vi "Create.vi"(8 "error in (no error)":errorcluster) -> (0 "error out":errorcluster, 3 "String Argument Matching Comparator":refnum<class "Matching String Input Comparator.lvclass">)   [LabVIEW 2020, in "Matching String Input Comparator.lvclass"]
uses:
  Matching String Input Comparator.lvclass
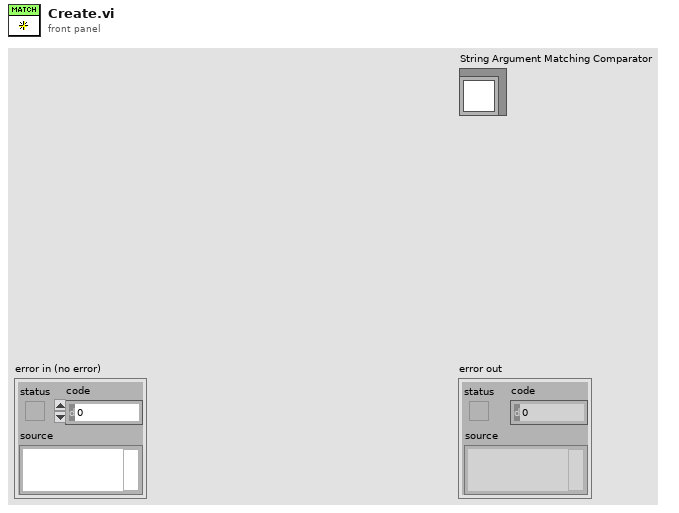
[diagram p1: front panel]
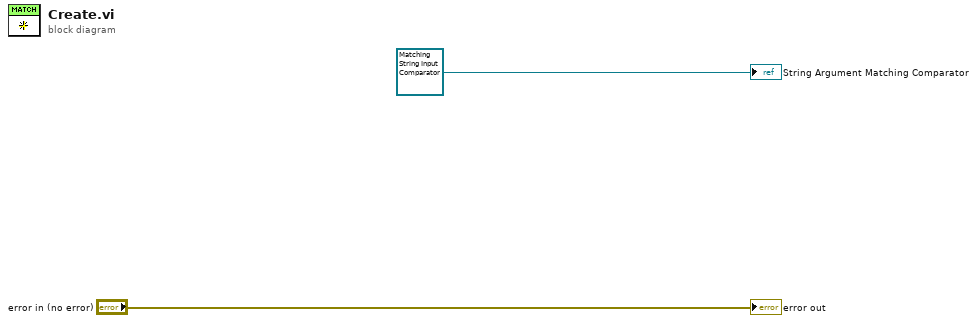
[diagram p0: block diagram]
diagram:
  "error out" <- "error in (no error)"
  "String Argument Matching Comparator" <- refnum<class "Matching String Input Comparator.lvclass"> refnum ("String Argument Matching Comparator")
